vi "BUFMGR_sendresponseBack.vi"(7 "error in (no error)":errorcluster, 9 "buffer":T3, 10 "Qname":string) -> ()   [LabVIEW 2016]
uses:
  private/vis/BufferStruct.ctl
panel:
  in  "buffer 2":T1
  in  "response struct":T2
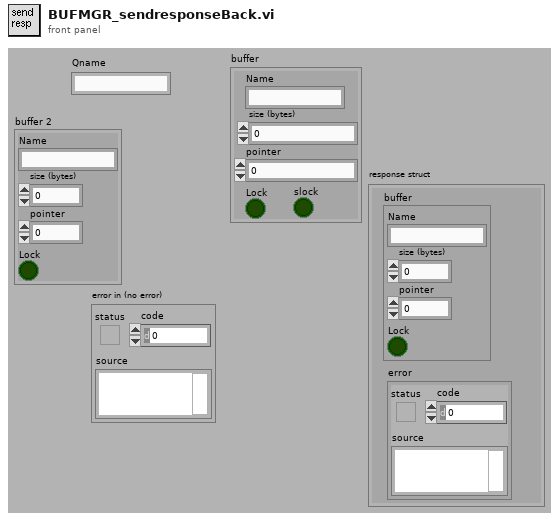
[diagram p1: front panel]
types:
  T1 = cluster{"Name":string, "size (bytes)":u64, "pointer":u64, "Lock":bool}
  T2 = cluster{"buffer":cluster{"Name":string, "size (bytes)":u64, "pointer":u64, "Lock":bool}, "error ":errorcluster}
  T3 = typedef "BufferStruct.ctl" = cluster{"Name":string, "size (bytes)":u64, "pointer":u64, "Lock":bool, "slock":bool}
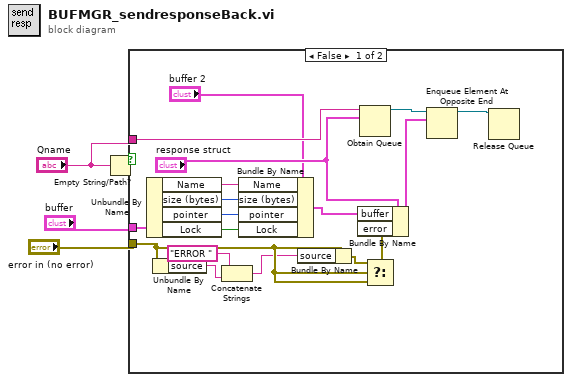
[diagram p0: block diagram]
diagram:
  n1 = Empty String/Path?(string/path="Qname") -> (empty?=w4:bool)
  n2 = case shown="False" w4 {
    tunnel: "buffer" -> [w11 _]
    tunnel: "error in (no error)" -> [w16 _]
    tunnel: "Qname" -> [w22 _]
    frame False {
      n3 = Unbundle By Name(w11) -> ("Name"=w10:string, "size (bytes)"=w7:u64, "pointer"=w8:u64, "Lock"=w9:bool)
      n4 = Unbundle By Name(w16) -> ("source"=w15:string)
      n5 = Concatenate Strings("ERROR " ("string"), w15) -> (w13:string)
      n6 = Bundle By Name(cluster="buffer 2", "Name"=w10, "size (bytes)"=w7, "pointer"=w8, "Lock"=w9) -> (w6:T1)
      n7 = Bundle By Name(cluster=w16, "source"=w13) -> (w12:errorcluster)
      n8 = Obtain Queue(name (unnamed)=w22, element data type="response struct") -> (queue out=w21:refnum<queue>)  [unwired: 3 in, 2 out]
      n9 = Select(t=w12, s=w16, f=w16) -> (s? t:f=w17:errorcluster)
      n10 = Bundle By Name(cluster="response struct", "buffer"=w6, "error"=w17) -> (w19:T2)
      n11 = Enqueue Element At Opposite End(queue=w21, element=w19) -> (queue out=w20:refnum<queue>)  [unwired: 1 in, 3 out]
      n12 = Release Queue(queue=w20) -> ()  [unwired: 1 in, 4 out]
    }
    frame True {
    }
  }
